vi "OriginTRJs.vi"(3 "file (use dialog)":path=path "C:/Lasermachining/Labviewprogram/gasjet/machinecapillary/singletrjwithconstantabrate/trj/basic.trj", 4 "Horizontal Line":T1={"Y-Offset"=-9.0, "Length"=9.0, "X-Offset"=25.5}, 5 "Vertical Line":T2={"X-Offset"=20.0, "Length"=7.0, "Y-Offset"=-8.5}) -> (1 "Startpoints":dbl[][](array[numeric]), 2 "TRJs":path[](array[path]))   [LabVIEW 2009]
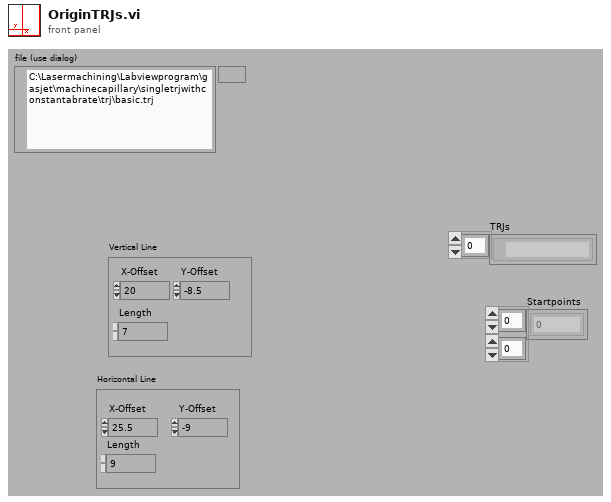
[diagram p1: front panel]
types:
  T1 = cluster{"Y-Offset":dbl, "Length":dbl, "X-Offset":dbl}
  T2 = cluster{"X-Offset":dbl, "Length":dbl, "Y-Offset":dbl}
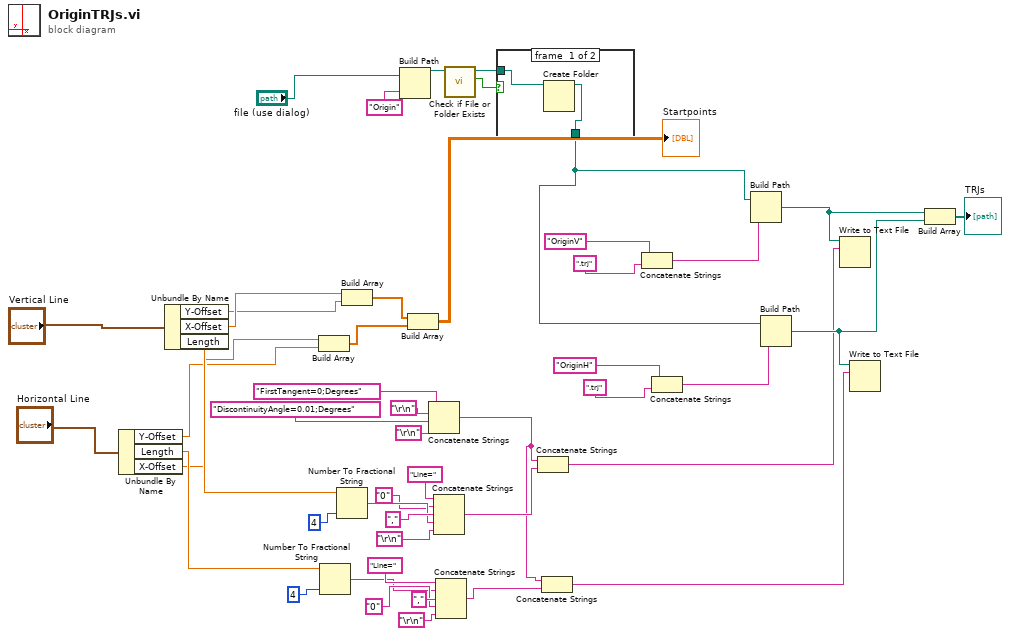
[diagram p0: block diagram]
diagram:
  n1 = Unbundle By Name("Horizontal Line") -> ("Y-Offset"=w7:dbl, "Length"=w23:dbl, "X-Offset"=w8:dbl)
  n2 = Unbundle By Name("Vertical Line") -> ("Y-Offset"=w9:dbl, "X-Offset"=w10:dbl, "Length"=w36:dbl)
  n3 = Build Array(w8, w7) -> (w16:dbl[])
  n4 = Number To Fractional String(number=w23, precision (6)=i16 4) -> (F-format string=w19:string)  [unwired: 1 in, 1 out]
  n5 = Number To Fractional String(number=w36, precision (6)=i16 4) -> (F-format string=w35:string)  [unwired: 1 in, 1 out]
  n6 = Build Array(w10, w9) -> (w17:dbl[])
  n7 = Build Path(base path="file (use dialog)", name or relative path="Origin") -> (appended path=w5:path)
  n8 = Build Array(w17, w16) -> (→"Startpoints":dbl[][])
  n9 = Concatenate Strings("FirstTangent=0;Degrees" ("string"), "\r\n", "DiscontinuityAngle=0.01;Degrees" ("string"), "\r\n") -> (w22:string)
  n10 = Concatenate Strings("Line=" ("string"), "0" ("string"), "," ("string"), w35, "\r\n") -> (w28:string)
  n11 = Concatenate Strings("Line=" ("string"), w19, "," ("string"), "0" ("string"), "\r\n") -> (w21:string)
  n12 = call <vilib>:"Check if File or Folder Exists.vi"("path"=w5) -> ("file or folder exists?"=w3:bool, "dup path"=w4:path)  [unwired: 8 in, 1 out]
  n13 = case shown="False" w3 {
    tunnel: w4 -> [w49 w50]
    tunnel: [w48 w50] -> w1
    frame #0 {
      n14 = Create Folder(path (use dialog)=w49) -> (created path=w48:path)  [unwired: 2 in, 2 out]
    }
    frame #1 {
    }
  }
  n15 = Concatenate Strings(w22, w28) -> (w15:string)
  n16 = Concatenate Strings(w22, w21) -> (w14:string)
  n17 = Concatenate Strings("OriginV" ("string"), ".trj" ("string")) -> (w38:string)
  n18 = Concatenate Strings("OriginH" ("string"), ".trj" ("string")) -> (w32:string)
  n19 = Build Path(base path=w1, name or relative path=w38) -> (appended path=w33:path)
  n20 = Build Path(base path=w1, name or relative path=w32) -> (appended path=w29:path)
  n21 = Write to Text File(file (use dialog)=w33, text=w15) -> ()  [unwired: 1 in, 4 out]
  n22 = Write to Text File(file (use dialog)=w29, text=w14) -> ()  [unwired: 1 in, 4 out]
  n23 = Build Array(w33, w29) -> (→"TRJs":path[])
